vi "Build Plot Names.vi"(4 "Plot Display Names":string[](array[string])) -> (1 "Consolidated Display Names":string[](array[string]))   [LabVIEW 2013]
uses:
  <userlib>/_OpenG.lib/string/string.llb/Trim Whitespace (String)__ogtk.vi
panel:
  out "x-y*floor(x/y)":i32
  in  "y":i32
  in  "X":i32
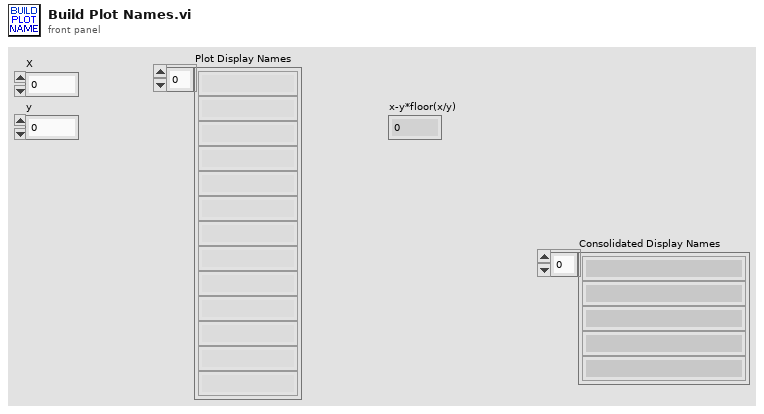
[diagram p1: front panel]
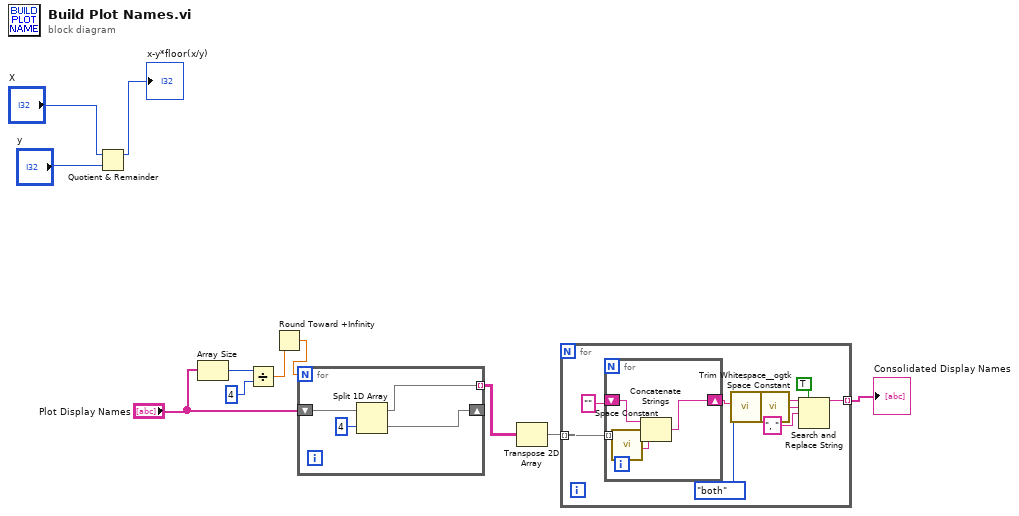
[diagram p0: block diagram]
diagram:
  n1 = Quotient & Remainder(x="X", y="y") -> (x-y*floor(x/y)=→"x-y*floor(x/y)":i32)  [unwired: 1 out]
  n2 = Array Size(array="Plot Display Names") -> (size(s)=w8:i32)
  n3 = Divide(x=w8, y=4 ("index")) -> (x/y=w6:dbl)
  n4 = Round Toward +Infinity(x=w6) -> (ceil(x): smallest int >= x=w5:dbl)
  n5 = for {
    N: w5 -> [_]
    shift-right: [w13] -> _
    shift-left: "Plot Display Names" -> [w14]
    tunnel: [w12] -> w3 mode=indexing
    n6 = Split 1D Array(array=w14, index=4) -> (first subarray=w12:string[], second subarray=w13:string[])
  }
  n7 = Transpose 2D Array(2D array=w3) -> (transposed array=w2:string[][])
  n8 = for {
    tunnel: w2 -> [w24] mode=indexing
    tunnel: [w16] -> w1 mode=indexing
    n9 = for {
      tunnel: w24 -> [w28] mode=indexing
      shift-right: [w26] -> w22
      shift-left: "" -> [w27]
      n10 = call <vilib>:"Space Constant.vi"() -> ("String"=w25:string)
      n11 = Concatenate Strings(w27, w28, w25) -> (w26:string)
    }
    n12 = call-poly <userlib>:"Trim Whitespace__ogtk.vi"("Remove (leading and trailing)"=enum16{"leading", "trailing", "both"}."both", "String in"=w22) -> ("String out"=w17:string)  [unwired: 5 in]
    n13 = call <vilib>:"Space Constant.vi"() -> ("String"=w19:string)
    n14 = Search and Replace String(replace all?=TRUE ("replace all? (F)"), input string=w17, search string=w19, replace string=", ") -> (result string=w16:string)  [unwired: 4 in, 3 out]
  }
  "Consolidated Display Names" <- w1
